vi "Write PWM.vi"(0 "Session Handle":T1, 5 "Max PWM":dbl format="%#_13g", 7 "Min PWM":dbl format="%#_13g", 11 "error in (no error)":errorcluster) -> (4 "Session Handle Out":T1, 15 "error out":errorcluster)   [LabVIEW 2015, in "Peltier.lvclass"]
uses:
  Peltier.lvclass
  Typedefs/Session Handle.ctl
  PAS/PAS.lvclass
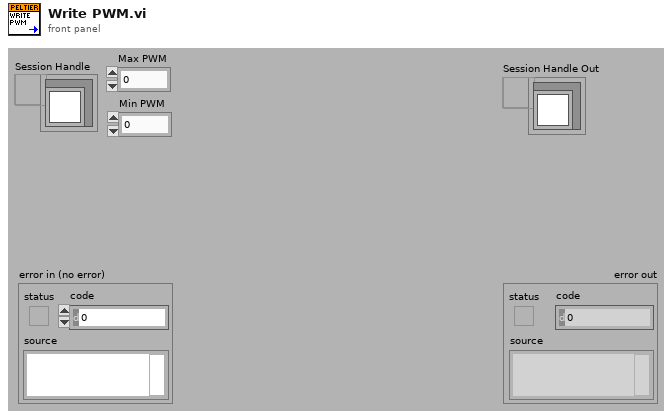
[diagram p1: front panel]
types:
  T1 = typedef "Peltier.lvclass/Session Handle.ctl" = refnum<data-value>
  T2 = typedef "XNET Frame CAN.ctl" = cluster{"timestamp":timestamp, "payload":u8[], "identifier":u32, "type":T3, "extended?":bool, "echo?":bool}
  T3 = typedef "XNET Frame Type CAN.ctl" = u8
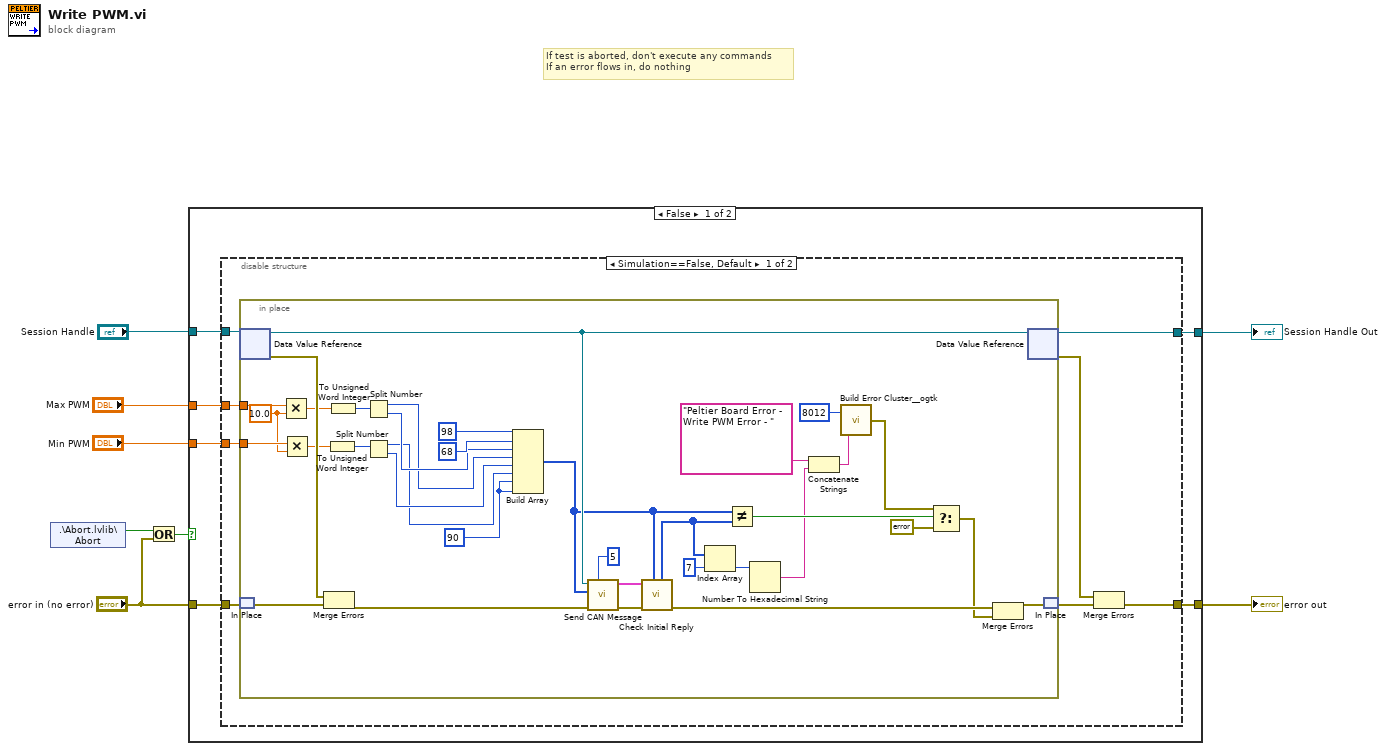
[diagram p0: block diagram]
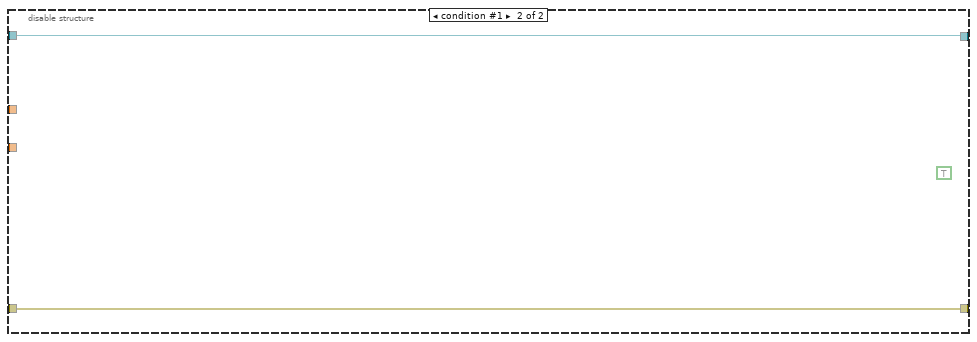
[diagram p2: hidden frame]
diagram:
  # "If test is aborted, don't execute any commands\nIf an error flows in, do nothing"
  n1 = shared-variable ".\\Abort.lvlib\\Abort"() -> (w7:bool)  [unwired: 1 in, 1 out]
  n2 = Or(x=w7, y="error in (no error)") -> (x .or. y?=w5:bool)
  n3 = case shown="False" w5 {
    tunnel: [w14 w61] -> w3
    tunnel: [w13 w60] -> w8
    tunnel: "Session Handle" -> [w12 w61]
    tunnel: "error in (no error)" -> [w11 w60]
    tunnel: "Max PWM" -> [w10 _]
    tunnel: "Min PWM" -> [w9 _]
    frame False {
      n4 = disable-structure shown="Simulation==False, Default" {
        disable-tunnel: [w22 w59] -> w14
        disable-tunnel: [w19 w58] -> w13
        disable-tunnel: w12 -> [w18 w59]
        disable-tunnel: w11 -> [w17 w58]
        disable-tunnel: w10 -> [w16 _]
        disable-tunnel: w9 -> [w15 _]
        frame condition #0 (active) {
          n5 = in-place {
            in-place-border: w16 -> [w37]
            in-place-border: w15 -> [w36]
            w26 = u8 90 ("new element/subarray")
            w35 = 10.0 ("y")
            n6 = in-place-dvr #1(w18) -> (w48:refnum<class "Peltier.lvclass">, w56:errorcluster)
            n7 = in-place-match #2(w17) -> (w55:errorcluster)
            n8 = Multiply(x=w37, y=w35) -> (x*y=w34:dbl)
            n9 = Multiply(x=w36, y=w35) -> (x*y=w33:dbl)
            n10 = Merge Errors(w56, w55) -> (w54:errorcluster)
            n11 = To Unsigned Word Integer(number=w33) -> (unsigned 16bit integer=w29:u16)
            n12 = To Unsigned Word Integer(number=w34) -> (unsigned 16bit integer=w32:u16)
            n13 = Split Number(x=w32) -> (hi(x)=w30:u8, lo(x)=w31:u8)
            n14 = Split Number(x=w29) -> (hi(x)=w27:u8, lo(x)=w28:u8)
            n15 = Build Array(u8 98 ("new element/subarray"), u8 68 ("new element/subarray"), w31, w30, w28, w27, w26, w26) -> (w47:u8[])
            n16 = call "Send CAN Message.vi"("Number of Retries"=5, "error in (no error)"=w54, "payload"=w47, "Peltier In"=w48) -> ("error out"=w25:errorcluster, "Reply"=w52:T2[])  [unwired: 5 in, 1 out]
            n17 = call "Check Initial Reply.vi"("Write Message"=w47, "error in (no error)"=w25, "Reply"=w52) -> ("error out"=w24:errorcluster, "Whole Payload"=w45:u8[])  [unwired: 5 in, 2 out]
            n18 = Index Array(array=w45, index=7) -> (element=w43:u8)
            n19 = Not Equal?(x=w47, y=w45) -> (x != y?=w46:bool)
            n20 = Number To Hexadecimal String(2:w43) -> (0:w41:string)  [unwired: 1 in]
            n21 = Concatenate Strings("Peltier Board Error - Write PWM Error - " ("string"), w41) -> (w40:string)
            n22 = call <userlib>:"Build Error Cluster__ogtk.vi"("String to Prepend to source (\"\")"=w40, "code"=8012) -> ("error out"=w50:errorcluster)
            n23 = Select(t=w50, s=w46, f=errorcluster {"status"=FALSE, "code"=0, "source"=""}) -> (s? t:f=w23:errorcluster)
            n24 = Merge Errors(w24, w23) -> (w57:errorcluster)
            n25 = in-place-dvr #1(w48) -> (w22:T1, w20:errorcluster)
            n26 = in-place-match #2(w57) -> (w21:errorcluster)
          }
          n27 = Merge Errors(w20, w21) -> (w19:errorcluster)
        }
        frame condition #1 {
          (unwired) TRUE
        }
      }
    }
    frame True {
    }
  }
  "error out" <- w8
  "Session Handle Out" <- w3
